vi "Set Ingredient.vi"(8 "error in (no error)":errorcluster, 10 "Ingredient":T1, 11 "Item Summary in":refnum<class "Item Summary.lvclass">) -> (0 "error out":errorcluster, 3 "Item Summary out":refnum<class "Item Summary.lvclass">)   [LabVIEW 2020, in "Item Summary.lvclass"]
uses:
  Item Summary.lvclass
  Item/Ingredient.ctl
  Item/Item.lvclass
  Item Summary.lvclass/Item Summary.ctl
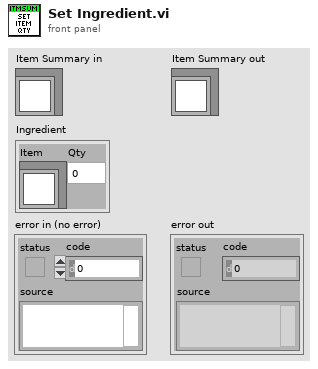
[diagram p1: front panel]
types:
  T1 = typedef "Item.lvclass/Ingredient.ctl" = cluster{"Item":refnum<class "Item.lvclass">, "Qty":dbl}
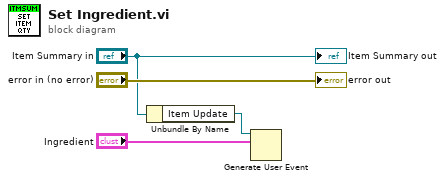
[diagram p0: block diagram]
diagram:
  n1 = Unbundle By Name("Item Summary in") -> ("Item Update"=w2:refnum<user-event>)
  n2 = Generate User Event(user event=w2, event data cluster="Ingredient") -> ()  [unwired: 2 in, 2 out]
  "error out" <- "error in (no error)"
  "Item Summary out" <- "Item Summary in"
